vi "updateStatus.vi"(8 "error in (no error)":errorcluster, 10 "tcpDevice":refnum<class "tcpDevice.lvclass">, 11 "deviceHeartbeat in":refnum<class "deviceHeartbeat.lvclass">) -> (0 "error out":errorcluster, 1 "status":T1, 2 "tcpDevice out":refnum<class "tcpDevice.lvclass">, 3 "deviceHeartbeat out":refnum<class "deviceHeartbeat.lvclass">, 4 "newValue":bool, 5 "timeout?":bool)   [LabVIEW 2016, in "deviceHeartbeat.lvclass"]
uses:
  deviceHeartbeat.lvclass
  typedefs/deviceStatus.ctl
  typedefs/statusEnum.ctl
  tcpDevice/tcpDevice.lvclass
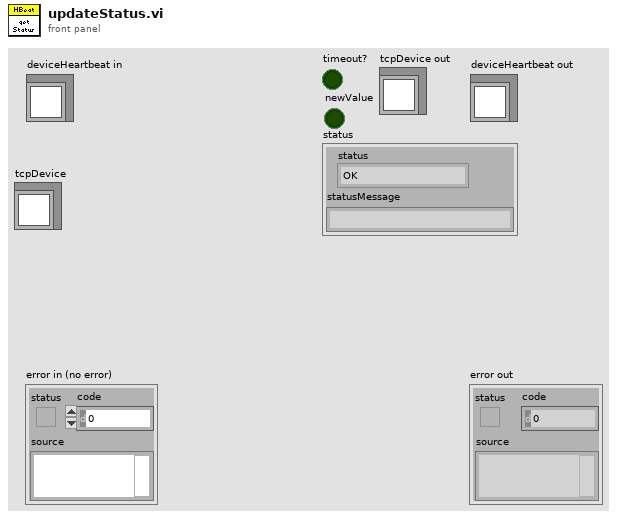
[diagram p1: front panel]
types:
  T1 = typedef "deviceStatus.ctl" = cluster{"status":T2, "statusMessage":string}
  T2 = typedef "statusEnum.ctl" = enum16{"OK", "TIMEOUT", "MSGERROR"}
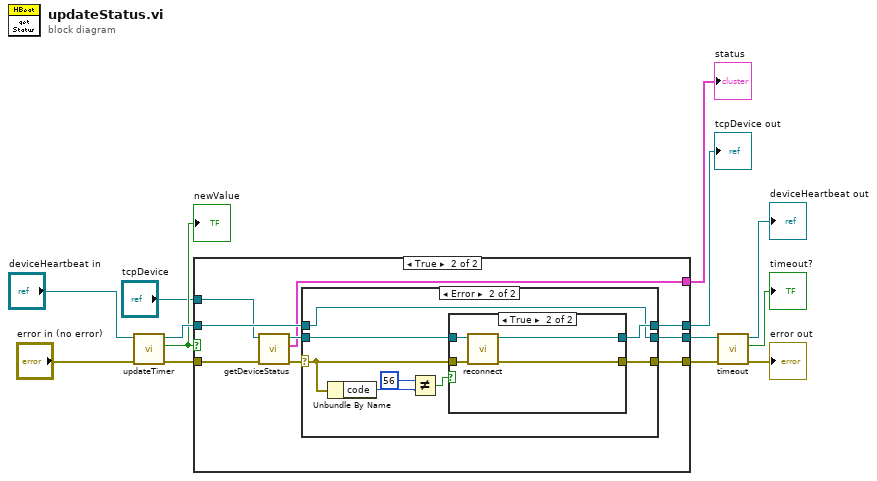
[diagram p0: block diagram]
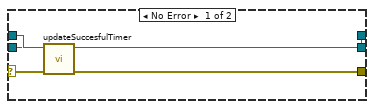
[diagram p3: hidden frame]
diagram:
  n1 = call "updateTimer.vi"("error in (no error)"="error in (no error)", "deviceHeartbeat in"="deviceHeartbeat in") -> ("error out"=w5:errorcluster, "getStatus?"=w4:bool, "deviceHeartbeat out"=w7:refnum<class "deviceHeartbeat.lvclass">)  [unwired: 7 in]
  "newValue" <- w4
  n2 = case shown="True" w4 {
    tunnel: [w15 w24] -> w10
    tunnel: [w16 w25] -> w11
    tunnel: w7 -> [w16 w23]
    tunnel: w5 -> [w15 w21]
    tunnel: [_ w17] -> w3
    tunnel: "tcpDevice" -> [w14 w20]
    tunnel: [w14 w18] -> w1
    frame False {
    }
    frame True {
      n3 = call-dynamic "getDeviceStatus.vi"("error in (no error)"=w21, "tcpDevice in"=w20) -> ("error out"=w22:errorcluster, "status"=w17:T1, "tcpDevice out"=w19:refnum<class "tcpDevice.lvclass">)  [unwired: 7 in]
      n4 = case shown="Error" w22 {
        selector: w22 -> [w27 w34]
        tunnel: [w29 w37] -> w24
        tunnel: w23 -> [w28 w35]
        tunnel: [w30 w35] -> w25
        tunnel: w19 -> [w26 w38]
        tunnel: [w26 w36] -> w18
        frame No Error {
          n5 = call "updateSuccesfulTimer.vi"("error in (no error)"=w27, "deviceHeartbeat in"=w28) -> ("error out"=w29:errorcluster, "deviceHeartbeat out"=w30:refnum<class "deviceHeartbeat.lvclass">)  [unwired: 8 in]
        }
        frame Error {
          n6 = Unbundle By Name(w34) -> ("code"=w33:i32)
          n7 = Not Equal?(x=56, y=w33) -> (x != y?=w32:bool)
          n8 = case shown="True" w32 {
            tunnel: w38 -> [w40 w44]
            tunnel: w34 -> [w39 w43]
            tunnel: [w39 w42] -> w37
            tunnel: [w40 w41] -> w36
            frame False {
              # "timeout doesn't need to re-connect"
            }
            frame True {
              n9 = call-dynamic "reconnect.vi"("error in (no error)"=w43, "tcpDevice in"=w44) -> ("error out"=w42:errorcluster, "tcpDevice out"=w41:refnum<class "tcpDevice.lvclass">)  [unwired: 8 in]
            }
          }
        }
      }
    }
  }
  "status" <- w3
  "tcpDevice out" <- w1
  n10 = call "timeout.vi"("error in (no error)"=w10, "deviceHeartbeat in"=w11) -> ("error out"=→"error out":errorcluster, "timeout?"=→"timeout?":bool, "deviceHeartbeat out"=→"deviceHeartbeat out":refnum<class "deviceHeartbeat.lvclass">)  [unwired: 7 in]
